vi "MeasurementServer_FourProbeMeasurement_WriteValue.vi"(0 "gRPCid":T3, 1 "FourProbeRawData":T1, 3 "error in (no error)":errorcluster) -> (10 "error out":errorcluster)   [LabVIEW 2019]
uses:
  build/Release/labview_measurement_server.dll
  MeasurementServer_gRPCid.ctl
  labview-grpc-measurement-server.lvlib
  MeasurementServer_ErrorOutData.ctl
  MeasurementServer_FourProbeRawData.ctl
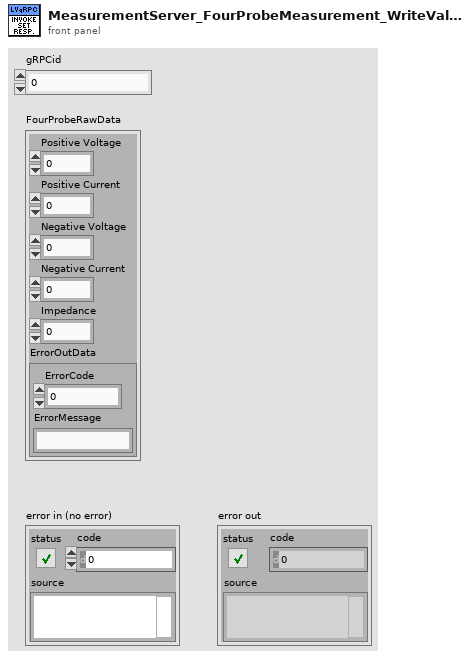
[diagram p1: front panel]
types:
  T1 = typedef "MeasurementServer_FourProbeRawData.ctl" = cluster{"Positive Voltage":sgl, "Positive Current":sgl, "Negative Voltage":sgl, "Negative Current":sgl, "Impedance":sgl, "ErrorOutData":T2}
  T2 = typedef "labview-grpc-measurement-server.lvlib/MeasurementServer_ErrorOutData.ctl" = cluster{"ErrorCode":i32, "ErrorMessage":string}
  T3 = typedef "labview-grpc-measurement-server.lvlib/MeasurementServer_gRPCid.ctl" = u64
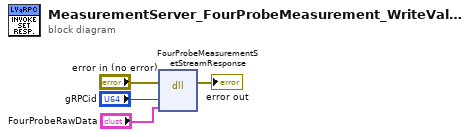
[diagram p0: block diagram]
diagram:
  n1 = dll-call lib="C:/Users/chericks/Desktop/OCV/labview-grpc-query-server/build/Release/labview_measurement_server.dll" fn="FourProbeMeasurementSetStreamResponse"(error in="error in (no error)", "id"="gRPCid", "data"="FourProbeRawData") -> (error out=→"error out":errorcluster)  [unwired: 5 in, 1 out]
